vi "Update Module Execution Status.vi"(8 "error in (no error)":errorcluster, 10 "Running?":bool, 11 "Module ID":i32=-1) -> (0 "error out":errorcluster)   [LabVIEW 2020, in "My Cloneable Module.lvlib"]
doc: "Fire the Get Module Execution Status request.\n_____\nCreated using Delacor QMH Event Scripter 3.0.0.12.\n_____\nBased on DQMH Project Template 6.0.0.91."
uses:
  My Cloneable Module.lvlib
  Get Module Execution Status Argument--cluster.ctl
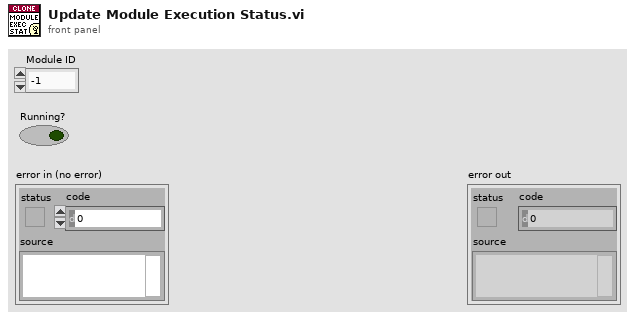
[diagram p1: front panel]
types:
  T1 = typedef "My Cloneable Module.lvlib/Get Module Execution Status Argument--cluster.ctl" = cluster{"Module ID":i32, "Running?":bool}
  T2 = typedef "My Cloneable Module.lvlib/Broadcast Events--cluster.ctl" = cluster{"Module Did Init":refnum<user-event>, "Status Updated":refnum<user-event>, "Error Reported":refnum<user-event>, "Did Something":refnum<user-event>, "Module Did Stop":refnum<user-event>, "Update Module Execution Status":refnum<user-event>}
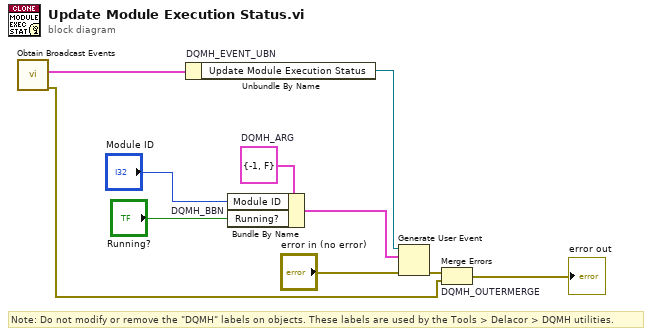
[diagram p0: block diagram]
diagram:
  w5 = T1 {"Module ID"=-1, "Running?"=FALSE}  # DQMH_ARG
  # "Note: Do not modify or remove the \"DQMH\" labels on objects. These labels are used by the Tools > Delacor > DQMH utilities."
  n1 = call "Obtain Broadcast Events.vi"() -> ("error out"=w2:errorcluster, "My Cloneable Module Broadcast Events"=w1:T2)  [unwired: 10 in]
  n2 = Unbundle By Name "DQMH_EVENT_UBN"(w1) -> ("Update Module Execution Status"=w7:refnum<user-event>)
  n3 = Bundle By Name "DQMH_BBN"(cluster=w5, "Module ID"="Module ID", "Running?"="Running?") -> (w8:T1)
  n4 = Generate User Event(user event=w7, event data cluster=w8, error in="error in (no error)") -> (error out=w6:errorcluster)  [unwired: 1 in, 1 out]
  n5 = Merge Errors "DQMH_OUTERMERGE"(w6, w2) -> (→"error out":errorcluster)
